vi "Aqu6009.vi"(8 "error in (no error)":errorcluster, 10 "timeout":dbl=1.0, 11 "Refnum in":refnum<k21>) -> (0 "error out":errorcluster, 1 "OK":bool, 2 "data 2":waveform(dbl)[](array[waveform]), 3 "Refnum out":refnum<k21>)   [LabVIEW 2011]
uses:
  DAQmx Fill In Error Info.vi
panel:
  out "x-y":u32
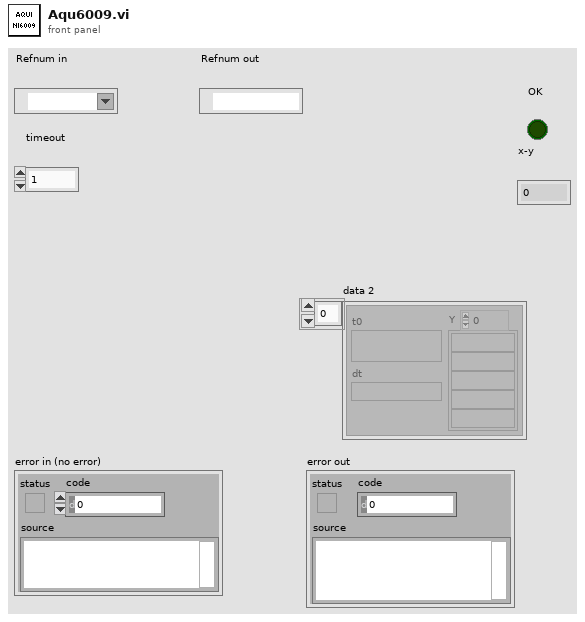
[diagram p1: front panel]
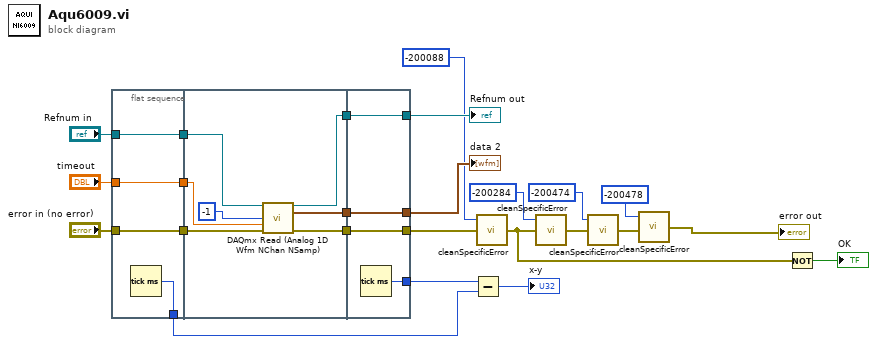
[diagram p0: block diagram]
diagram:
  n1 = flat-sequence {
    tunnel: "Refnum in" -> [w26]
    tunnel: "timeout" -> [w27]
    tunnel: "error in (no error)" -> [w28]
    tunnel: [w28] -> w17
    tunnel: [w27] -> w16
    tunnel: [w26] -> w15
    tunnel: [w25] -> w10
    tunnel: w17 -> [w33]
    tunnel: w16 -> [w32]
    tunnel: w15 -> [w30]
    tunnel: [w35] -> w14
    tunnel: [w34] -> w13
    tunnel: [w31] -> w12
    tunnel: [w37] -> w23
    tunnel: [w38] -> w6
    tunnel: [w39] -> w24
    tunnel: w14 -> [w39]
    tunnel: w13 -> [w38]
    tunnel: w12 -> [w37]
    tunnel: [w36] -> w11
    frame #0 {
      n2 = Tick Count (ms)() -> (millisecond timer value=w25:u32)
    }
    frame #1 {
      n3 = call "DAQmx Read (Analog 1D Wfm NChan NSamp).vi"("task/channels in"=w30, "number of samples per channel"=-1, "timeout"=w32, "error in"=w33) -> ("task out"=w31:refnum<k21>, "data"=w35:waveform(dbl)[], "error out"=w34:errorcluster)  [unwired: 9 in]
    }
    frame #2 {
      n4 = Tick Count (ms)() -> (millisecond timer value=w36:u32)
    }
  }
  n5 = Subtract(x=w11, y=w10) -> (x-y=→"x-y":u32)
  n6 = call "cleanSpecificError.vi"("error out"=w6, "error code"=-200088) -> ("error IO"=w2:errorcluster)  [unwired: 2 in, 1 out]
  n7 = call "cleanSpecificError.vi"("error out"=w2, "error code"=-200284 ("code")) -> ("error IO"=w19:errorcluster)  [unwired: 2 in, 1 out]
  n8 = call "cleanSpecificError.vi"("error out"=w19, "error code"=-200474 ("code")) -> ("error IO"=w5:errorcluster)  [unwired: 2 in, 1 out]
  n9 = call "cleanSpecificError.vi"("error out"=w5, "error code"=-200478 ("code")) -> ("error IO"=→"error out":errorcluster)  [unwired: 2 in, 1 out]
  n10 = Not(x=w2) -> (.not. x?=→"OK":bool)
  "data 2" <- w24
  "Refnum out" <- w23
